vi "send.vi"(0 "HGF_Notifier":refnum<class "HGF_Notifier.lvclass">, 2 "Object":refnum<class>, 3 "timeout in ms (-1)":i32, 5 "error in (no error)":errorcluster, 9 "mode (Queue)":bool) -> (14 "dup HGF_Notifier":refnum<class "HGF_Notifier.lvclass">, 17 "timed out?":bool, 19 "error out":errorcluster)   [LabVIEW 2014, in "HGF_BaseClasses.lvlib" / "HGF_Notifier.lvclass"]
doc: "Send an object.\n\nHint: This is a dynamic dispatch VI to be implemented by the child class."
uses:
  HGF_Notifier.lvclass
  HGF_Auxiliary/HGF_Auxiliary.lvlib
  HGF_Auxiliary/Severity.ctl
  HGF_Auxiliary/ErrorCode.ctl
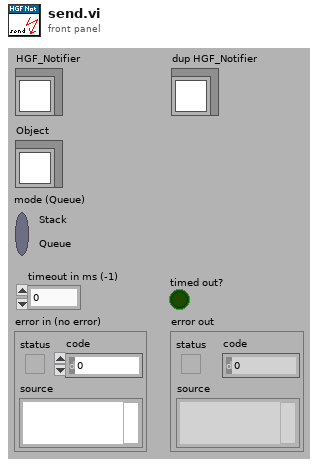
[diagram p1: front panel]
types:
  T1 = typedef "HGF_Auxiliary.lvlib/ErrorCode.ctl" = enum32{"No error", "Function not supported.", "This VI is for friends only.", "Reference object aready exisits.", "Parameter out of range.", "Not a rendezvous.", "Invalid notifier reference.", "Invalid queue reference.", "Self-Test not supported.", "Reset not supported.", "IDN query not supported.", "Error query not supported.", "Incorrect addressee.", "Object already exists.", "No class name specified", "Driver not supported", "Attribute is not writable"}
  T2 = typedef "HGF_Auxiliary.lvlib/Severity.ctl" = enum16{"Info", "Warning", "Fault", "Error", "Fatal"}
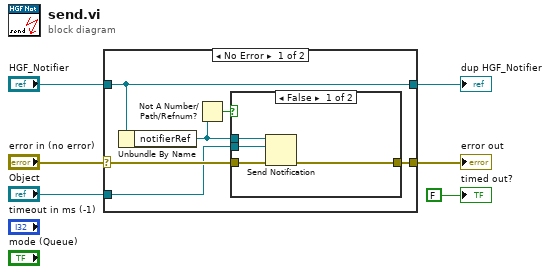
[diagram p0: block diagram]
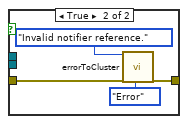
[diagram p2: hidden frame]
diagram:
  n1 = case shown="No Error" "error in (no error)" {
    selector: "error in (no error)" -> [w11 w21]
    tunnel: [w12 w22] -> w6
    tunnel: "HGF_Notifier" -> [w12 w22]
    tunnel: [w10 w21] -> w3
    tunnel: "Object" -> [w9 _]
    frame No Error {
      n2 = Unbundle By Name(w12) -> ("notifierRef"=w8:refnum<notifier>)
      n3 = Not A Number/Path/Refnum?(number/path/refnum=w8) -> (NaN/Path/Refnum?=w7:bool)
      n4 = case shown="False" w7 {
        tunnel: w8 -> [w16 _]
        tunnel: w11 -> [w15 w19]
        tunnel: [w14 w20] -> w10
        tunnel: w9 -> [w13 _]
        frame False {
          n5 = Send Notification(notification=w13, notifier=w16, error in (no error)=w15) -> (error out=w14:errorcluster)  [unwired: 1 out]
        }
        frame True {
          n6 = call "errorToCluster.vi"("error code"=ErrorCode."Invalid notifier reference." ("HGF_Error"), "error in (no error)"=w19, "severity (Error)"=Severity."Error") -> ("error out"=w20:errorcluster)  [unwired: 2 in, 14 out]
        }
      }
    }
    frame Error {
    }
  }
  "error out" <- w3
  "dup HGF_Notifier" <- w6
  "timed out?" <- FALSE ("timed out?")
